vi "PW_LDA wrapper_PN.vi"(0 "PW_LDA control cluster":T2={"Block data directory"=path "C:/LDAPW data/x=140, y=0.79 10ms", "An samp. rate (Hz)"=5000.0, "PW sampling rate (Hz)"=10.0, "PW samples per block"=300, "High threshold (V)"=2.5, "An. data prefix"="Analogue_", "LDA data prefix"="LDA_", "PW data prefix"="PW_", "LDA arr. t. prefix"="LDA_arr_t_", "filename suffix"=".txt", "interp. method"=1, "PW hardware delay (s)"=0.00085, "PW timing TOF fraction (0..1)"=0.5, "- LDA V"=TRUE, "PW TOF prefix"="PW_TOF_", "- LDA U"=FALSE, "- PW"=FALSE, "format"="%.16f"} {"interp. method" items=["nearest", "linear", "spline", "cubic Hermite", "Lagrange"]}, 1 "Wrapper controls":T1={"N blocks"=20, "PW lag time start (s)"=0.0, "PW lag time finish (s)"=0.0, "PW lag time dt (s)"=0.002, "Desired lag time for stats (s)"=0.0, "stats order"=4, "PDF(T) or hist(F)"=TRUE, "Nbins U"=32, "Nbins V"=32, "Mean shift"=FALSE, "2nd comp."="v"}, 2 "Y pos":dbl) -> (13 "Y pos array":dbl[](array[numeric]), 14 "PW reverse flow factor":dbl=0.4096244131455399 format="%#_12g", 15 "All checksums okay":bool=TRUE, 16 "PW timeout fraction":dbl=0.012743125419181758, 17 "Rlag (m)":dbl[](array[numeric]), 18 "PW TOFmin cutoff fraction":dbl=0.001006036217303823, 19 "tlag (s)":dbl[](array[numeric]), 20 "Corr coeff. tau, U with PW lag time":dbl[](array[numeric])=[0.5572999061568849], 21 "Corr coeff. tau, V with PW lag time":dbl[](array[numeric])=[0.004298805974359152], 22 "Corr coeff. tau, UV with PW lag time":dbl[](array[numeric])=[-0.027234703441453165], 23 "Un-weighted stats":dbl[](array[numeric])=[0.43858590934936287, 0.0001041533801020402, 0.1463894386367247, -0.02457196354778752, 0.14225051082889828, -0.032883046319648, 0.02271213590005001, -0.030848260891795806, 0.020839430073599775, 1.6419504590373541, -0.017474933147796762, 0.26978335280499277, -0.029543622581726194, 0.2945426390265555, 0.03238576446532323, -0.16519945715490864, 0.09286281865203916, -0.1935441070795655, 0.050985700918232096, 6.779683511945926, -0.08550977449408034, 1.3778799507125228, -0.057532383884902095, 1.7073049444938453], 24 "Weighted stats":dbl[](array[numeric])=[0.29100923404306667, 0.003216404163501678, 0.14065168910394837, -0.0247339603407455, 0.13448157508469313, -0.024361823150874228, 0.02659079325503093, -0.029636337396151475, 0.03772631974230529, 1.334444078744411, -0.011181958349287136, 0.21516440173044252, -0.028718928576858992, 0.22755186986970175, 0.28082969747599357, -0.11371827995167888, 0.13120158382958494, -0.14829498580423525, 0.15080960131183163, 4.836358465323817, -0.08045155436100758, 0.9592749415988219, -0.10674333693310743, 1.117860734806738], 25 "Sync'd stats":dbl[](array[numeric])=[9.99808755719511, 0.30885001488943276, 0.007197594295384736, 0.0008830575291785714, 0.0942694270166445, -0.008369791241477553, 0.060882863617426265, -0.01639558282333675, 0.010021524505129425, -0.01919225938374916, -0.0007955532121171695, 1.081048634581646, -0.011113747117756345, 0.12842502593386193, 0.008713818152611364, 0.12343248218360064, 0.08560249872100657, -0.07896455364935291, 0.015579535060437296, -0.11211030347834718, -0.061338520775783154, 3.042693307359604, -0.042626691321700154, 0.4955635209260197, 0.12378215036474391, 0.6595145821544666, 4.519172989851708e-05, 5.91346531093378e-05, -0.00017430143164649768, -0.00021527961324126435, 0.019839799313372736, -0.000509583419996228, 0.002759758803593956, 0.0003530448602341623, 0.0027055215355820342, 0.0029382422465524904, -0.0014638561896802816, -0.00014761963473996917, -0.0025406145666271576, -0.0022637148963733722, 0.06455947587270858, -0.0015743835544541394, 0.012668430780602572, 0.004325247318679681, 0.016824152878582684, 0.025106752706962183, -0.015875686245146146, -0.006475981348485304, -0.02739532903645526, -0.026953861773836463, 0.0011723340448017852, -3.987256514453876e-05, 0.0001817240280323321, 3.3680352685292565e-06, 0.0001497262646277783, 0.0001415833115273109, -2.4675085527676877e-05, -1.8809858479403676e-05, -8.088971584500279e-05, -0.00010100909182132213, 0.002614922297046162, -9.514408147817417e-05, 0.000557542035268452, 0.00016469969685146263, 0.000676633068557077, 0.0008384732237052391, -0.0005110951840304789, -0.00037365314293173524, -0.0010324578366570894, -0.001198305036722039, 0.013265366110818869, 0.0002711809483820985, 0.0041643047012696185, 0.002418010535035754, 0.006215671063356672, 1.1217352583572477e-05, 6.344155160186447e-08, -7.664065504136946e-07, -2.129897917839301e-06, -5.306341303367024e-06, 0.0001195173198309039, -4.245802227303591e-06, 2.746649310552381e-05, 7.569471202211092e-06, 3.2191154509505075e-05, 1.0249380040762277e-05, -1.7041287981748652e-05, -2.1627786768005314e-05, -4.264139397480935e-05, -5.809335881508808e-05, 0.0005797512887398283, 3.959658308454404e-06, 0.00019648014213266728, 0.00010700455589582494, 0.00028675676203472286, 0.00018623104770989905, -0.0002861767092517544, -0.0002737802435507171, -0.0005887639922204611, -0.0007158972853763932, 1.6151006536221114e-05, -9.955295514799653e-07, 2.3778438821819195e-06, 3.3595543391506415e-07, 2.0535496541026416e-06, -5.444039236573482e-06, 3.5020997050138697e-07, -1.3997177108814566e-06, -1.6719714892314103e-06, -3.015766572187203e-06, 4.2187949113226374e-05, -1.9755684504406396e-06, 1.0753467015735944e-05, 4.47680139746371e-06, 1.4534458720814612e-05, -8.658088459848207e-06, -9.520921055642612e-06, -1.4596272866351805e-05, -2.6395769780853278e-05, -3.5099628626523324e-05, 0.0002370235802228167, 1.4637476763147469e-05, 0.00010148850801440133, 7.029378841714576e-05, 0.00016132576692576137], 26 "Total pre-sync LDA points":i32=44933, 27 "Total sync'd points":i32=5964)   [LabVIEW 2011]
uses:
  PW_LDA control cluster.ctl
  PW_LDA wrapper control cluster.ctl
  <vilib>/gmath/NI_Gmath.lvlib
  <vilib>/Analysis/NI_AALBase.lvlib
  <vilib>/Analysis/NI_AALPro.lvlib
panel:
  in  "Precision":i16=16
  out "PW lag time":dbl
  out "LDA V":dbl[](array[numeric])
  out "LDA U":dbl[](array[numeric])
  in  "Write lagged correls. file?":bool
  out "tlag(s) Rlag(m) tauU tauV tauUV":string="0.0000000000000000\t0.0000000000000000\t0.5572999061568848\t0.0042988059743592\t-0.0272347034414532\r\n"
  out "Lag time loop no.":i32=1
  out "Lag time loops to do":i32=1
  out "Block time pulse checksums":bool[](array[boolean])=[TRUE, TRUE, TRUE, TRUE, TRUE, TRUE, TRUE, TRUE, TRUE, TRUE, TRUE, TRUE, TRUE, TRUE, TRUE, TRUE, TRUE, TRUE, TRUE, TRUE]
  in  "Write raw numbers to file?":bool
  out "LDA orig. and sync'd U,V phase plot":cluster{"all rows":dbl[], "all rows":dbl[]}[](graph)
  out "PW, LDA_U, V, UV phase plot":cluster{"first row":dbl[], "yi":dbl[]}[](graph)
  out "Curr. block no.":i32=20
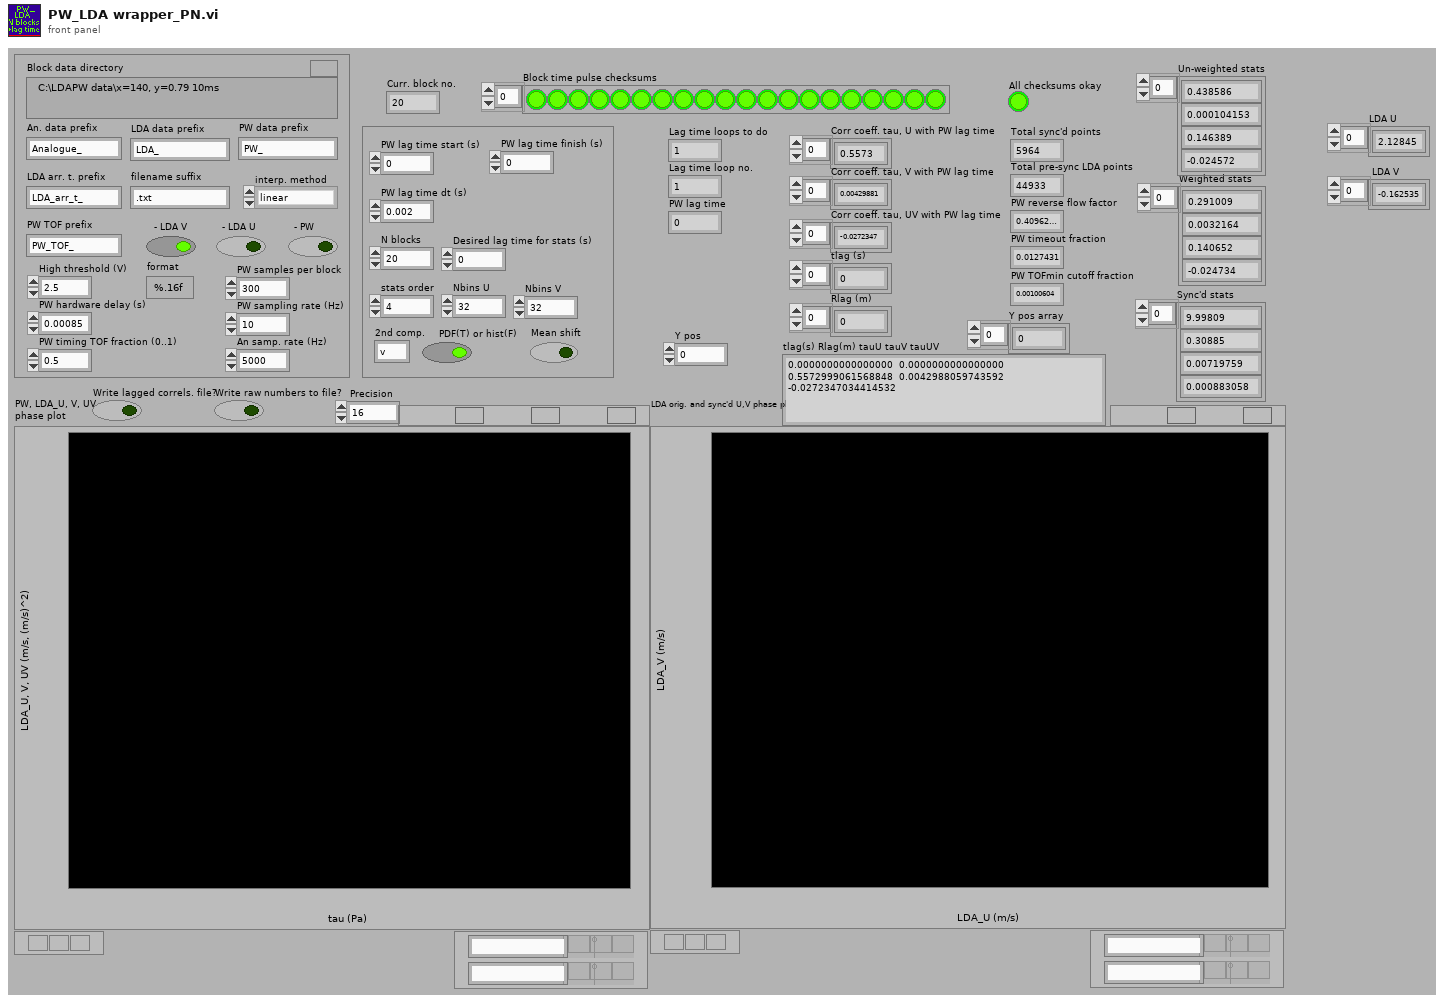
[diagram p1: front panel]
types:
  T1 = typedef "PW_LDA wrapper control cluster.ctl" = cluster{"N blocks":i32, "PW lag time start (s)":dbl, "PW lag time finish (s)":dbl, "PW lag time dt (s)":dbl, "Desired lag time for stats (s)":dbl, "stats order":i32, "PDF(T) or hist(F)":bool, "Nbins U":i32, "Nbins V":i32, "Mean shift":bool, "2nd comp.":string}
  T2 = typedef "PW_LDA control cluster.ctl" = cluster{"Block data directory":path, "An samp. rate (Hz)":dbl, "PW sampling rate (Hz)":dbl, "PW samples per block":i32, "High threshold (V)":dbl, "An. data prefix":string, "LDA data prefix":string, "PW data prefix":string, "LDA arr. t. prefix":string, "filename suffix":string, "interp. method":i32, "PW hardware delay (s)":dbl, "PW timing TOF fraction (0..1)":dbl, "- LDA V":bool, "PW TOF prefix":string, "- LDA U":bool, "- PW":bool, "format":string}
  T3 = enum16{"open", "replace", "create", "open or create", "replace or create", "replace or create with confirmation"}
  T4 = cluster{"sync'd LDA U":dbl[], "sync'd LDA U":dbl[]}
  T5 = cluster{"sync'd LDA U":dbl[], "sync'd LDA U":dbl[]}[]
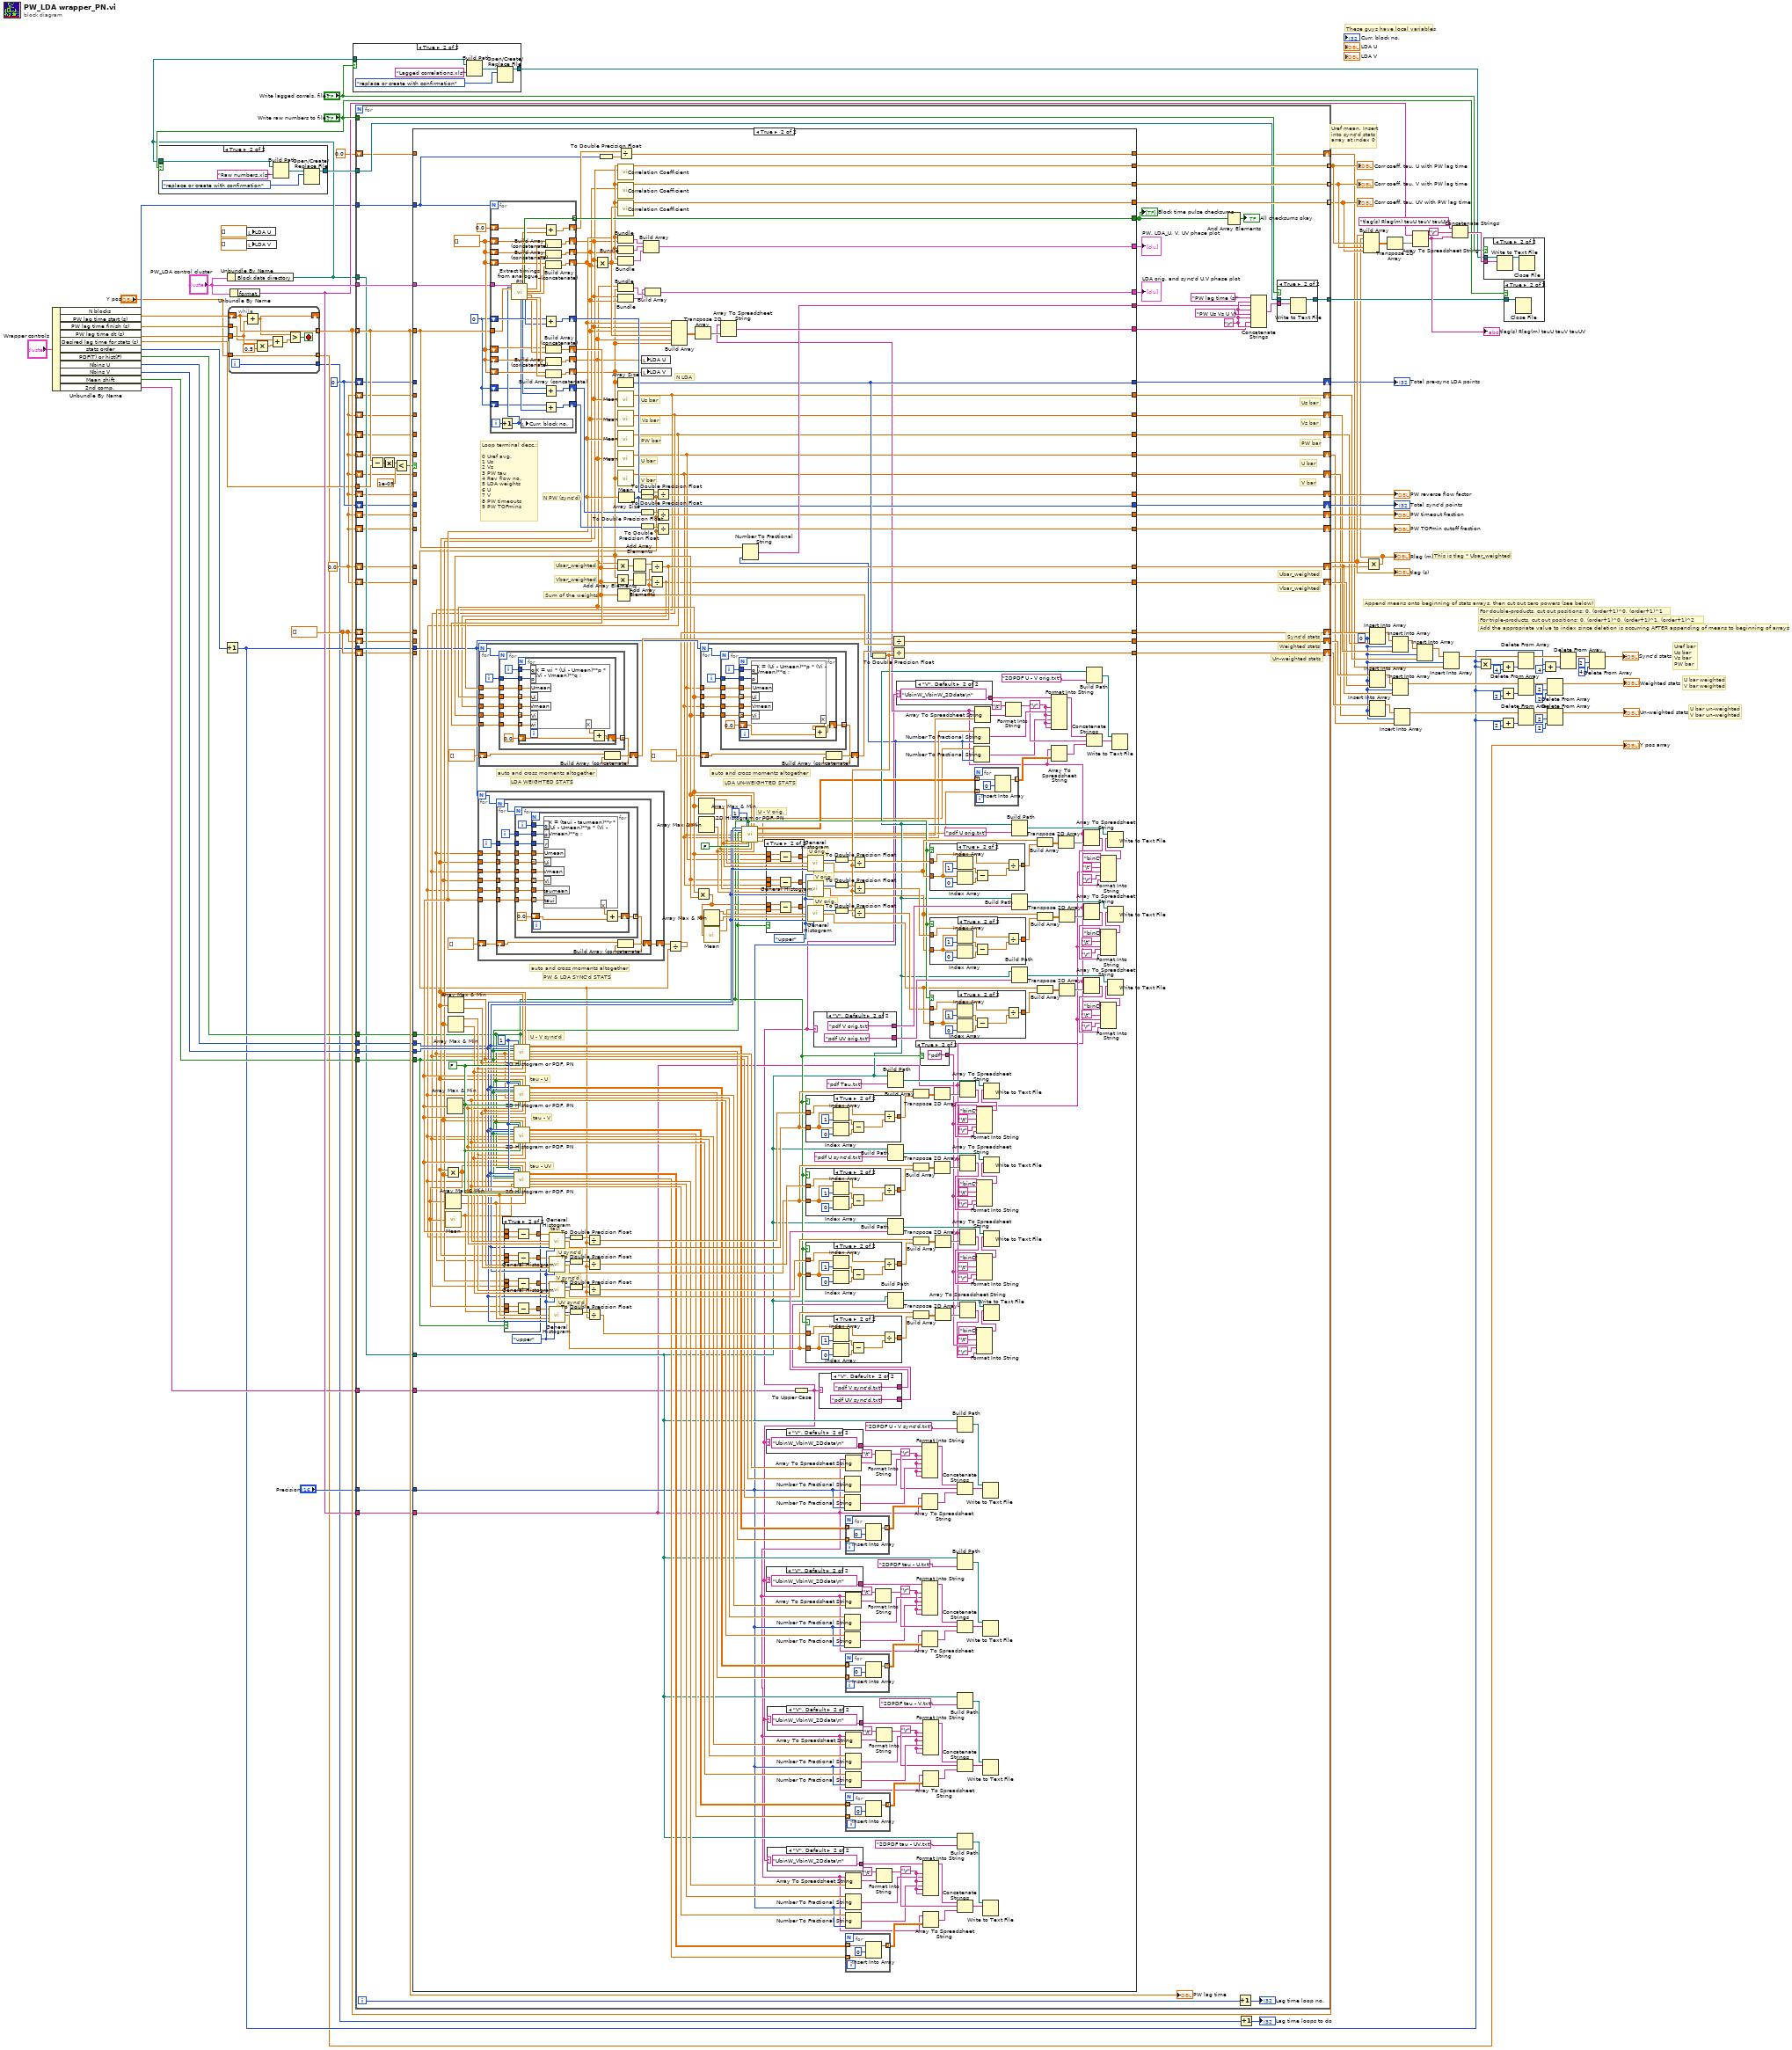
[diagram p0: block diagram]
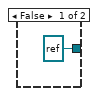
[diagram p3: hidden frame]
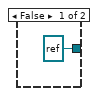
[diagram p4: hidden frame]
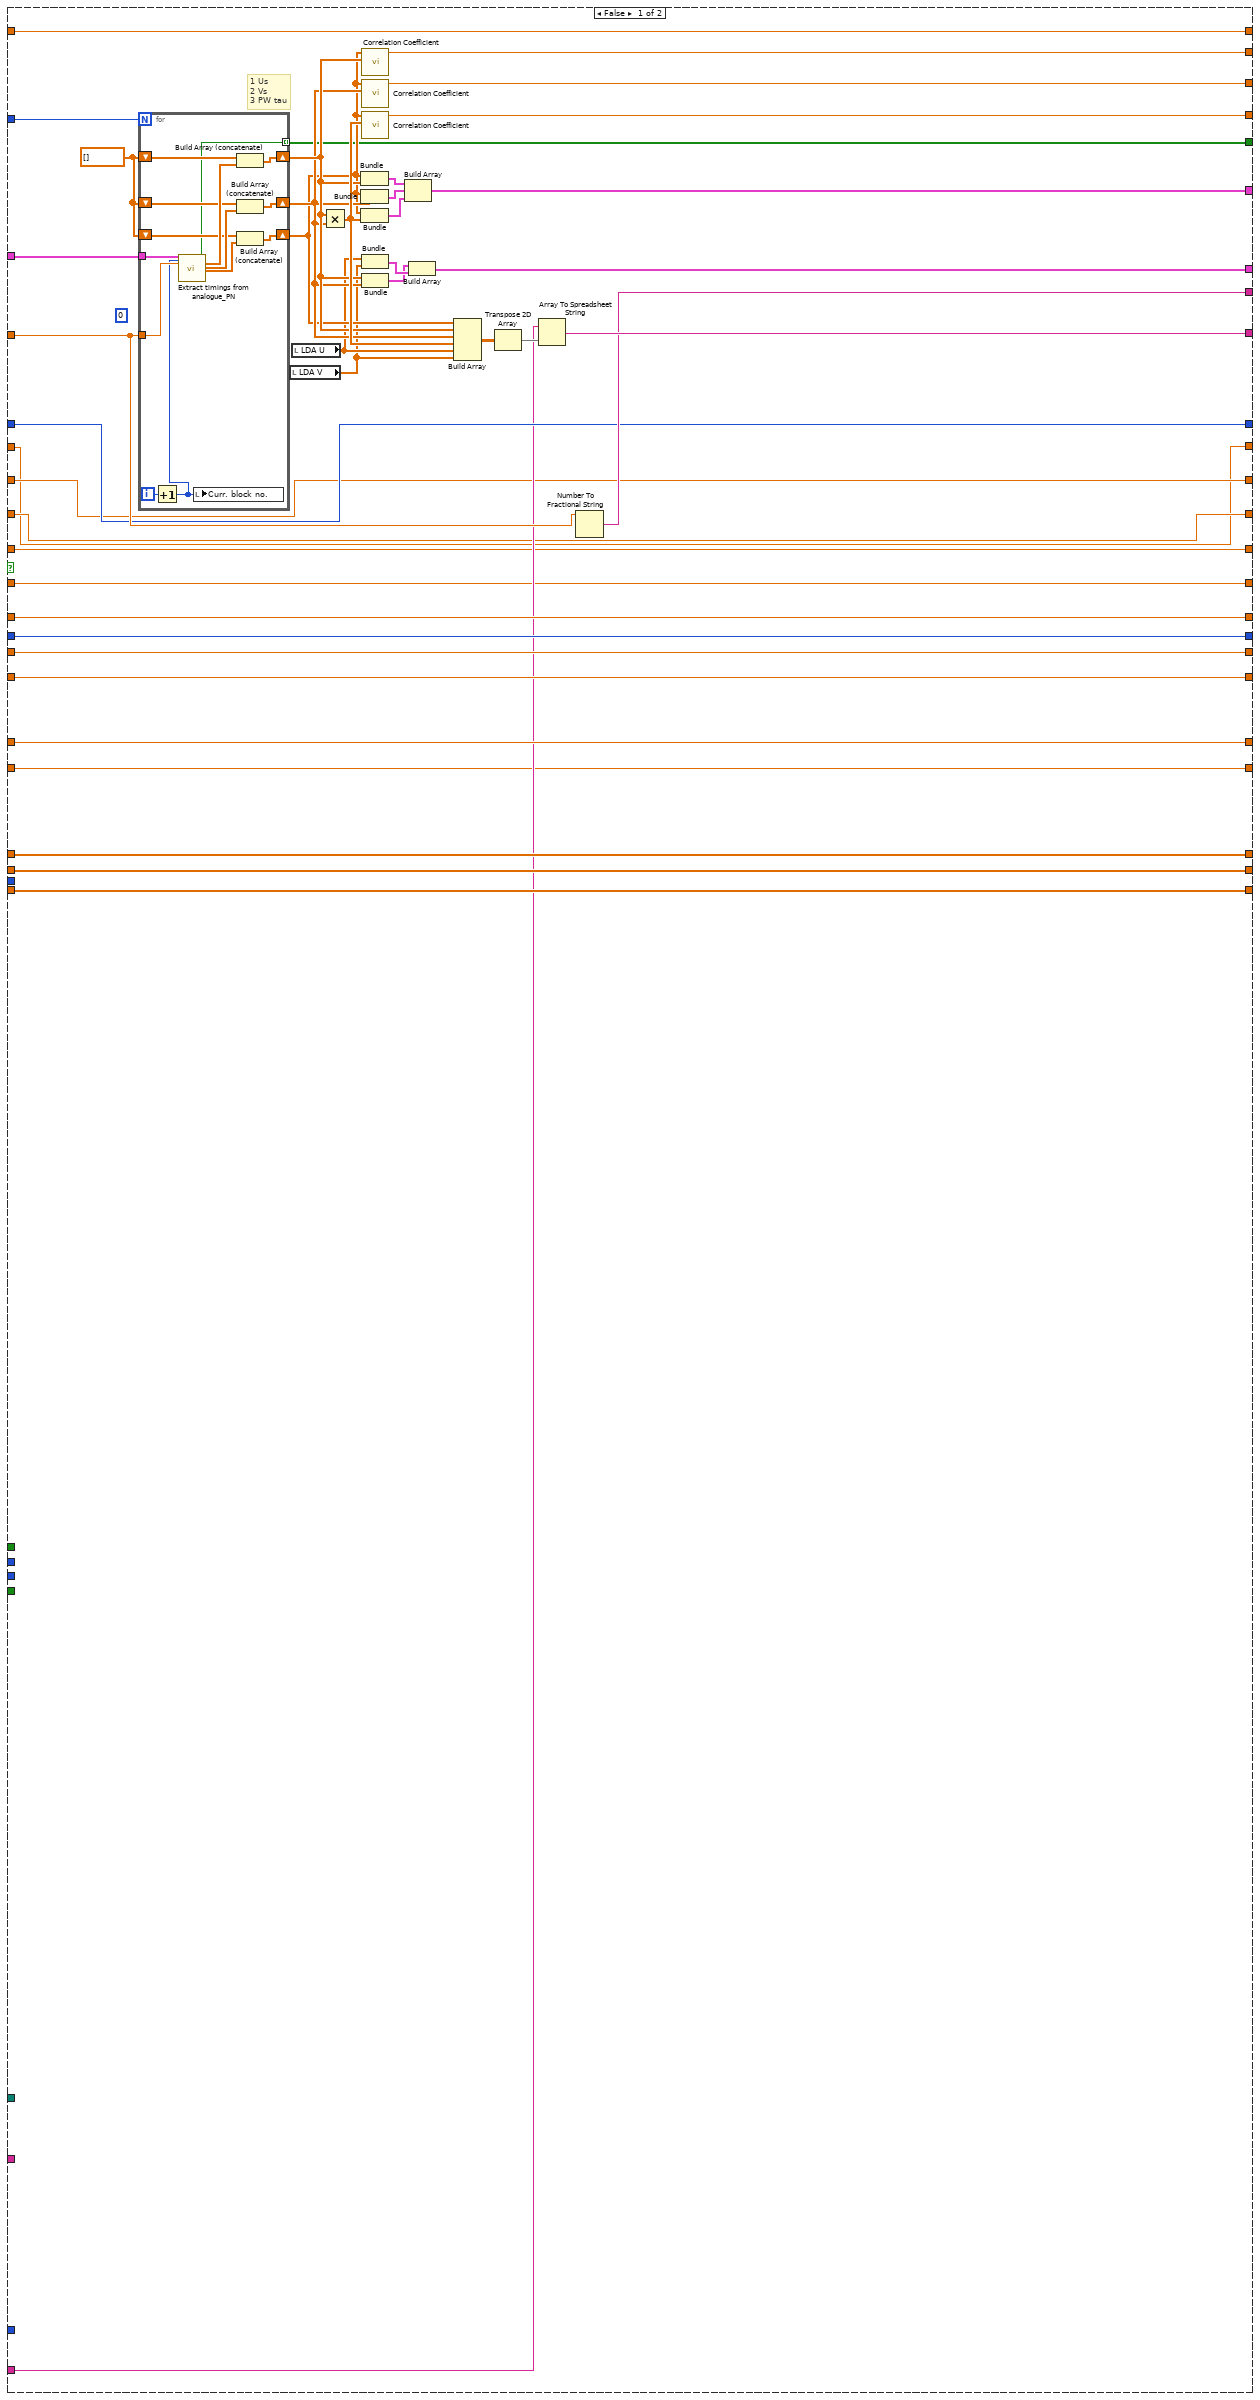
[diagram p7: hidden frame]
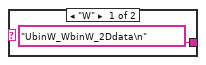
[diagram p8: hidden frame]
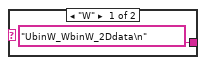
[diagram p9: hidden frame]
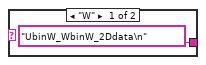
[diagram p10: hidden frame]
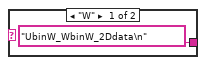
[diagram p11: hidden frame]
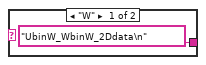
[diagram p12: hidden frame]
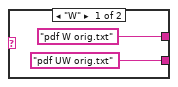
[diagram p13: hidden frame]
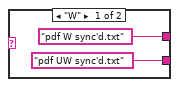
[diagram p18: hidden frame]
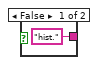
[diagram p19: hidden frame]
diagram:
  w5 = 0 ("index")
  w74 = dbl[] []
  w69 = 0
  w63 = 0.0
  # "Uref mean. Insert into sync'd stats array at index 0"
  # "Add the appropriate value to index since deletion is occurring AFTER appending of means to beginning of arrays"
  # "For triple-products, cut out positions: 0, (order+1)^0, (order+1)^1, (order+1)^2"
  # "For double-products, cut out positions: 0, (order+1)^0, (order+1)^1"
  # "U bar un-weighted\nV bar un-weighted"
  # "U bar weighted\nV bar weighted"
  # "Uref bar\nUs bar\nVs bar\nPW bar"
  # "Append means onto beginning of stats arrays, then cut out zero powers (see below)"
  # "This is tlag * Ubar_weighted"
  # "These guys have local variables"
  n1 = Unbundle By Name("Wrapper controls") -> ("N blocks"=w44:i32, "PW lag time start (s)"=w47:dbl, "PW lag time finish (s)"=w46:dbl, "PW lag time dt (s)"=w45:dbl, "Desired lag time for stats (s)"=w43:dbl, "stats order"=w37:i32, "PDF(T) or hist(F)"=w42:bool, "Nbins U"=w41:i32, "Nbins V"=w40:i32, "Mean shift"=w39:bool, "2nd comp."=w38:string)
  n2 = Increment(x=w37) -> (x+1=w12:i32)
  n3 = Unbundle By Name("PW_LDA control cluster") -> ("Block data directory"=w64:path)
  n4 = case shown="True" "Write raw numbers to file?" {
    tunnel: [refnum<file> refnum ("refnum out") w94] -> w82
    tunnel: w64 -> [_ w92]
    frame False {
    }
    frame True {
      n5 = Build Path(base path=w92, name or relative path="Raw numbers.xls") -> (appended path=w93:path)
      n6 = Open/Create/Replace File(file path (use dialog)=w93, operation (0:open)=T3."replace or create with confirmation") -> (refnum out=w94:refnum<file>)  [unwired: 1 in, 5 out]
    }
  }
  n7 = while {
    tunnel: w46 -> [w99]
    tunnel: w45 -> [w101]
    shift-right: [w103] -> _
    shift-left: w47 -> [w105]
    tunnel: [w105] -> w76 mode=indexing
    tunnel: [w104] -> w1
    tunnel: "Y pos" -> [w97]
    tunnel: [w97] -> w10 mode=indexing
    i -> [w104]
    stop <- w106 stop-if-true
    n8 = Add(x=w105, y=w101) -> (x+y=w103:dbl)
    n9 = Multiply(x=w101, y=0.5) -> (x*y=w100:dbl)
    n10 = Add(x=w99, y=w100) -> (x+y=w98:dbl)
    n11 = Greater?(x=w103, y=w98) -> (0:w106:bool)
  }
  "tlag (s)" <- w76
  "Y pos array" <- w10
  n12 = Unbundle By Name("PW_LDA control cluster") -> ("format"=w66:string)
  n13 = local write "LDA U"(dbl[] [] ("LDA U")) -> ()
  n14 = local write "LDA V"(dbl[] [] ("LDA V")) -> ()
  n15 = case shown="True" "Write lagged correls. file?" {
    tunnel: [refnum<file> refnum ("refnum out") w110] -> w80
    tunnel: w64 -> [_ w108]
    frame False {
    }
    frame True {
      n16 = Build Path(base path=w108, name or relative path="Lagged correlations.xls") -> (appended path=w109:path)
      n17 = Open/Create/Replace File(file path (use dialog)=w109, operation (0:open)=T3."replace or create with confirmation") -> (refnum out=w110:refnum<file>)  [unwired: 1 in, 5 out]
    }
  }
  n18 = for {
    tunnel: w44 -> [w179]
    tunnel: w76 -> [w164] mode=indexing
    tunnel: "Write raw numbers to file?" -> [w167]
    tunnel: [w178] -> w90 mode=indexing
    tunnel: [w177] -> w89 mode=indexing
    tunnel: [w176] -> w88 mode=indexing
    tunnel: w82 -> [w166]
    tunnel: [w168] -> w79
    tunnel: "PW_LDA control cluster" -> [w165]
    tunnel: w43 -> [w162]
    tunnel: w12 -> [w157]
    tunnel: w40 -> [w156]
    tunnel: w39 -> [w155]
    tunnel: w42 -> [w154]
    tunnel: w41 -> [w153]
    tunnel: w64 -> [w150]
    tunnel: "Precision" -> [w149]
    shift-right: [w158] -> w51
    shift-left: w63 -> [w143]
    shift-right: [w148] -> w61
    shift-left: w74 -> [w140]
    shift-right: [w147] -> w59
    shift-left: w74 -> [w139]
    shift-right: [w146] -> w56
    shift-left: w74 -> [w141]
    shift-right: [w152] -> w71
    shift-left: w63 -> [w135]
    shift-right: [w151] -> w70
    shift-left: w63 -> [w136]
    shift-right: [w142] -> w68
    shift-left: w69 -> [w132]
    shift-right: [w138] -> w73
    shift-left: w63 -> [w133]
    shift-right: [w137] -> w72
    shift-left: w69 -> [w134]
    tunnel: w66 -> [w131]
    shift-right: [w130] -> w54
    shift-left: w63 -> [w120]
    shift-right: [w129] -> w62
    shift-left: w63 -> [w121]
    shift-right: [w128] -> w53
    shift-left: w63 -> [w122]
    shift-right: [w127] -> w49
    shift-left: w63 -> [w123]
    shift-right: [w126] -> w50
    shift-left: w63 -> [w124]
    shift-right: [w125] -> w52
    shift-left: w63 -> [w118]
    tunnel: w38 -> [w119]
    shift-right: [w116] -> w4
    shift-left: 0.0 -> [w115]
    i -> [w114]
    w171 = "\r"
    # "Un-weighted stats"
    # "Weighted stats"
    # "Sync'd stats"
    # "Vbar_weighted"
    # "Ubar_weighted"
    # "V bar"
    # "U bar"
    # "PW bar"
    # "Vs bar"
    # "Us bar"
    n19 = Subtract(x=w164, y=w162) -> (x-y=w163:dbl)
    n20 = Absolute Value(x=w163) -> (abs(x)=w161:dbl)
    n21 = Less?(x=w161, y=1e-09) -> (x < y?=w159:bool)
    n22 = case shown="True" w159 {
      tunnel: w179 -> [w225 w241]
      tunnel: [w213 w526] -> w178
      tunnel: [w212 w525] -> w177
      tunnel: [w211 w524] -> w176
      tunnel: w164 -> [w204 w512]
      tunnel: [w209 w515] -> w117
      tunnel: [w192 w506] -> w142
      tunnel: [w193 w516] -> w138
      tunnel: [w194 w498] -> w137
      tunnel: [w197 w508] -> w147
      tunnel: [w208 w514] -> w170
      tunnel: [w207 w513] -> w169
      tunnel: w165 -> [w203 w511]
      tunnel: [w199 w507] -> w146
      tunnel: [w200 w505] -> w158
      tunnel: w157 -> [_ w497]
      tunnel: [w198 w396] -> w148
      tunnel: w156 -> [_ w472]
      tunnel: w155 -> [_ w458]
      tunnel: w154 -> [_ w335]
      tunnel: w153 -> [_ w473]
      tunnel: [w195 w489] -> w152
      tunnel: [w196 w488] -> w151
      tunnel: w150 -> [_ w265]
      tunnel: w149 -> [_ w259]
      tunnel: [w202 w258] -> w145
      tunnel: [w201 w257] -> w144
      tunnel: w143 -> [w200 _]
      tunnel: w141 -> [w199 _]
      tunnel: w140 -> [w198 _]
      tunnel: w139 -> [w197 _]
      tunnel: w136 -> [w196 _]
      tunnel: w135 -> [w195 _]
      tunnel: w134 -> [w194 _]
      tunnel: w133 -> [w193 _]
      tunnel: w132 -> [w192 _]
      tunnel: w131 -> [w191 w254]
      tunnel: [w185 w253] -> w130
      tunnel: [w186 w252] -> w129
      tunnel: [w187 w251] -> w128
      tunnel: [w188 w250] -> w127
      tunnel: [w189 w249] -> w126
      tunnel: [w190 w248] -> w125
      tunnel: w124 -> [w189 _]
      tunnel: w123 -> [w188 _]
      tunnel: w122 -> [w187 _]
      tunnel: w121 -> [w186 _]
      tunnel: w120 -> [w185 _]
      tunnel: w119 -> [_ w247]
      tunnel: w118 -> [w190 _]
      tunnel: [w184 w240] -> w116
      tunnel: w115 -> [w184 _]
      frame False {
        (unwired) 0 ("PW reverse flow samples")
        w210 = dbl[] [] ("sync'd LDA U")
        # "1 Us\n2 Vs\n3 PW tau"
        n23 = for {
          N: w225 -> [_]
          shift-right: [w236] -> w216
          shift-left: w210 -> [w238]
          shift-right: [w235] -> w215
          shift-left: w210 -> [w233]
          shift-right: [w232] -> w214
          shift-left: w210 -> [w230]
          tunnel: w204 -> [w227]
          tunnel: [w229] -> w209 mode=indexing
          tunnel: w203 -> [w228]
          i -> [w239]
          n24 = Increment(x=w239) -> (x+1=w226:i32)
          n25 = call "Extract timings from analogue_PN.vi"("PW_LDA control cluster"=w228, "Block no."=w226, "PW lag time (s)"=w227) -> ("valid bursts checksum status"=w229:bool, "sync'd LDA U"=w237:dbl[], "sync'd LDA V"=w234:dbl[], "PW tau"=w231:dbl[])  [unwired: 12 in, 9 out]
          n26 = local write "Curr. block no."(w226) -> ()
          n27 = Build Array (concatenate)(w238, w237) -> (w236:dbl[])
          n28 = Build Array (concatenate)(w233, w234) -> (w235:dbl[])
          n29 = Build Array (concatenate)(w230, w231) -> (w232:dbl[])
        }
        n30 = local read "LDA V"() -> (w205:dbl[])
        n31 = local read "LDA U"() -> (w206:dbl[])
        n32 = Multiply(x=w216, y=w215) -> (x*y=w217:dbl[])
        n33 = Bundle("sync'd LDA U"=w214, "sync'd LDA U"=w216) -> (w224:T4)  [unwired: 1 out]
        n34 = Bundle("sync'd LDA U"=w214, "sync'd LDA U"=w215) -> (w223:T4)  [unwired: 1 out]
        n35 = Bundle("sync'd LDA U"=w214, w217) -> (w222:cluster{"sync'd LDA U":dbl[], dbl[]})  [unwired: 1 out]
        n36 = call <vilib>:"Correlation Coefficient.vi"("Y"=w216, "X"=w214) -> ("correlation coefficient r"=w213:dbl)  [unwired: 9 out]
        n37 = call <vilib>:"Correlation Coefficient.vi"("Y"=w215, "X"=w214) -> ("correlation coefficient r"=w212:dbl)  [unwired: 9 out]
        n38 = call <vilib>:"Correlation Coefficient.vi"("Y"=w217, "X"=w214) -> ("correlation coefficient r"=w211:dbl)  [unwired: 9 out]
        n39 = Bundle("LDA U"=w206, "LDA V"=w205) -> (w221:cluster{"LDA U":dbl[], " LDA V":dbl[]})  [unwired: 1 out]
        n40 = Bundle("sync'd LDA U"=w216, "sync'd LDA U"=w215) -> (w220:T4)  [unwired: 1 out]
        n41 = Build Array(w224, w223, w222) -> (w202:T5)
        n42 = Build Array(w220, w221) -> (w201:cluster{"LDA U":dbl[], " LDA V":dbl[]}[])
        n43 = Build Array(w214, w216, w215, w217, w206, w205) -> (w219:dbl[][])
        n44 = Transpose 2D Array(2D array=w219) -> (transposed array=w218:dbl[][])
        n45 = Array To Spreadsheet String(array=w218, 3:w191) -> (spreadsheet string=w208:string)  [unwired: 1 out]
        n46 = Number To Fractional String(number=w204) -> (F-format string=w207:string)  [unwired: 3 out]
      }
      frame True {
        w476 = enum32{"lower", "upper"}."upper" ("inclusion")
        w479 = enum32{"lower", "upper"}."upper" ("inclusion")
        w276 = "\r"
        w296 = "\r"
        w306 = "\r"
        w332 = "\r"
        w343 = "\r"
        w495 = FALSE ("Interactive graph")
        w496 = 1 ("No. of blocks")
        w494 = 0 ("PW reverse flow samples")
        w523 = dbl[] [] ("sync'd LDA U")
        # "Sum of the weights"
        # "N PW (sync'd)"
        # "V bar"
        # "U bar"
        # "PW bar"
        # "Vs bar"
        # "Us bar"
        # "N LDA"
        # "UV orig."
        # "V orig."
        # "U orig."
        # "UV sync'd"
        # "V sync'd"
        # "U sync'd"
        # "tau"
        # "U - V orig."
        # "tau - UV"
        # "tau - V"
        # "tau - U"
        # "U - V sync'd"
        # "auto and cross moments altogether"
        # "auto and cross moments altogether"
        # "PW & LDA SYNC'd STATS"
        # "LDA UN-WEIGHTED STATS"
        # "LDA WEIGHTED STATS"
        # "Vbar_weighted"
        # "Ubar_weighted"
        # "auto and cross moments altogether"
        # "Loop terminal desc.:\n\n0 Uref avg.\n1 Us\n2 Vs\n3 PW tau\n4 Rev flow no.\n5 LDA weights\n6 U\n7 V\n8 PW timeouts\n9 PW TOFmins"
        n47 = for {
          N: w241 -> [_]
          shift-right: [w797] -> w465
          shift-left: w523 -> [w799]
          shift-right: [w796] -> w463
          shift-left: w523 -> [w794]
          shift-right: [w793] -> w467
          shift-left: w523 -> [w791]
          shift-right: [w790] -> w256
          shift-left: w523 -> [w789]
          shift-right: [w787] -> w255
          shift-left: w523 -> [w785]
          tunnel: w512 -> [w776]
          tunnel: [w784] -> w515 mode=indexing
          shift-right: [w782] -> w510
          shift-left: w523 -> [w781]
          shift-right: [w780] -> w518
          shift-left: w494 -> [w778]
          tunnel: w511 -> [w777]
          shift-right: [w772] -> w490
          shift-left: w494 -> [w770]
          shift-right: [w771] -> w491
          shift-left: w494 -> [w769]
          shift-right: [w767] -> w242
          shift-left: 0.0 -> [w766]
          i -> [w800]
          n48 = Increment(x=w800) -> (x+1=w774:i32)
          n49 = call "Extract timings from analogue_PN.vi"("PW_LDA control cluster"=w777, "Block no."=w774, "PW lag time (s)"=w776) -> ("No. of PW <TOFmin"=w773:i32, "Uref block avg."=w768:dbl, "No. of PW timeouts"=w775:i32, "valid bursts checksum status"=w784:bool, "PW reverse flow samples"=w779:i32, "sync'd LDA U"=w798:dbl[], "sync'd LDA V"=w795:dbl[], "PW tau"=w792:dbl[], "LDA weights"=w783:dbl[], "LDA U"=w788:dbl[], "LDA V"=w786:dbl[])  [unwired: 12 in, 2 out]
          n50 = local write "Curr. block no."(w774) -> ()
          n51 = Add(x=w766, y=w768) -> (x+y=w767:dbl)
          n52 = Add(x=w778, y=w779) -> (x+y=w780:i32)
          n53 = Add(x=w770, y=w775) -> (x+y=w772:i32)
          n54 = Add(x=w769, y=w773) -> (x+y=w771:i32)
          n55 = Build Array (concatenate)(w799, w798) -> (w797:dbl[])
          n56 = Build Array (concatenate)(w794, w795) -> (w796:dbl[])
          n57 = Build Array (concatenate)(w791, w792) -> (w793:dbl[])
          n58 = Build Array (concatenate)(w781, w783) -> (w782:dbl[])
          n59 = Build Array (concatenate)(w789, w788) -> (w790:dbl[])
          n60 = Build Array (concatenate)(w785, w786) -> (w787:dbl[])
        }
        n61 = Multiply(x=w465, y=w463) -> (x*y=w461:dbl[])
        n62 = Array Max & Min(array=w461) -> (max value=w477:dbl, min value=w478:dbl)  [unwired: 2 out]
        n63 = call <vilib>:"Mean.vi"("X"=w461) -> ("mean"=w459:dbl)  [unwired: 1 out]
        n64 = Array Max & Min(array=w467) -> (max value=w485:dbl, min value=w484:dbl)  [unwired: 2 out]
        n65 = Array Max & Min(array=w465) -> (max value=w482:dbl, min value=w483:dbl)  [unwired: 2 out]
        n66 = Array Max & Min(array=w463) -> (max value=w480:dbl, min value=w481:dbl)  [unwired: 2 out]
        n67 = Multiply(x=w465, y=w463) -> (x*y=w527:dbl[])
        n68 = To Double Precision Float(number=w241) -> (double precision float=w243:dbl)
        n69 = Multiply(x=w256, y=w510) -> (x*y=w522:dbl[])
        n70 = Multiply(x=w255, y=w510) -> (x*y=w519:dbl[])
        n71 = Add Array Elements(numeric array=w510) -> (sum=w509:dbl)
        n72 = Bundle("sync'd LDA U"=w467, "sync'd LDA U"=w465) -> (w534:T4)  [unwired: 1 out]
        n73 = Bundle("sync'd LDA U"=w467, "sync'd LDA U"=w463) -> (w533:T4)  [unwired: 1 out]
        n74 = Bundle("sync'd LDA U"=w467, w527) -> (w532:cluster{"sync'd LDA U":dbl[], dbl[]})  [unwired: 1 out]
        n75 = Divide(x=w242, y=w243) -> (x/y=w240:dbl)
        n76 = call <vilib>:"Correlation Coefficient.vi"("Y"=w465, "X"=w467) -> ("correlation coefficient r"=w526:dbl)  [unwired: 9 out]
        n77 = call <vilib>:"Correlation Coefficient.vi"("Y"=w463, "X"=w467) -> ("correlation coefficient r"=w525:dbl)  [unwired: 9 out]
        n78 = call <vilib>:"Correlation Coefficient.vi"("Y"=w527, "X"=w467) -> ("correlation coefficient r"=w524:dbl)  [unwired: 9 out]
        n79 = Bundle("sync'd LDA U"=w256, "sync'd LDA U"=w255) -> (w531:T4)  [unwired: 1 out]
        n80 = Bundle("sync'd LDA U"=w465, "sync'd LDA U"=w463) -> (w530:T4)  [unwired: 1 out]
        n81 = Array Size(array=w255) -> (size(s)=w506:i32)
        n82 = call <vilib>:"Mean.vi"("X"=w465) -> ("mean"=w253:dbl)  [unwired: 1 out]
        n83 = call <vilib>:"Mean.vi"("X"=w463) -> ("mean"=w252:dbl)  [unwired: 1 out]
        n84 = call "2D Histogram or PDF, PN.vi"("Nbins U"=w473, "Nbins V"=w472, "Mean shift"=w458, "Umean"=w253, "Vmean"=w252, "Umax"=w482, "No. of blocks"=w496, "Umin"=w483, "PDF"=w335, "Interactive graph"=w495, "V"=w463, "Vmax"=w480, "U"=w465, "Vmin"=w481) -> ("2D histogram or PDF"=w338:dbl[][], "U bin centre vals."=w339:dbl[], "V bin centre vals."=w340:dbl[], "UbinWidth"=w337:dbl, "VbinWidth"=w336:dbl)  [unwired: 1 out]
        n85 = call <vilib>:"Mean.vi"("X"=w467) -> ("mean"=w251:dbl)  [unwired: 1 out]
        n86 = for {
          N: w497 -> [w675]
          shift-right: [w673] -> w499
          shift-left: dbl[] [] -> [w674]
          tunnel: w467 -> [w672]
          tunnel: w251 -> [w671]
          tunnel: w465 -> [w670]
          tunnel: w463 -> [w669]
          tunnel: w253 -> [w668]
          tunnel: w252 -> [w667]
          i -> [w666]
          n87 = for {
            N: w675 -> [w680]
            tunnel: w670 -> [w687]
            tunnel: w669 -> [w686]
            tunnel: w667 -> [w685]
            tunnel: w668 -> [w684]
            shift-right: [w682] -> w673
            shift-left: w674 -> [w683]
            tunnel: w666 -> [w679]
            tunnel: w672 -> [w677]
            tunnel: w671 -> [w676]
            i -> [w678]
            n88 = for {
              N: w680 -> [_]
              tunnel: w684 -> [w698]
              tunnel: w687 -> [w697]
              tunnel: [w692] -> w681 mode=indexing
              tunnel: w685 -> [w695]
              tunnel: w686 -> [w694]
              tunnel: w678 -> [w693]
              tunnel: w679 -> [w691]
              tunnel: w677 -> [w690]
              tunnel: w676 -> [w689]
              i -> [w688]
              n89 = for {
                tunnel: w698 -> [w710]
                tunnel: w697 -> [w709] mode=indexing
                shift-right: [w707] -> w692
                shift-left: 0.0 -> [w706]
                tunnel: w688 -> [w703]
                tunnel: w695 -> [w705]
                tunnel: w694 -> [w704] mode=indexing
                tunnel: w693 -> [w702]
                tunnel: w691 -> [w701]
                tunnel: w690 -> [w700] mode=indexing
                tunnel: w689 -> [w699]
                n90 = formula code="X = (taui - taumean)**r * (Ui - Umean)**p * (Vi - Vmean)**q ;"("Umean"=w710, "Ui"=w709, "p"=w702, "Vi"=w704, "Vmean"=w705, "q"=w703, "r"=w701, "taumean"=w699, "taui"=w700) -> ("X"=w708:dbl)
                n91 = Add(x=w708, y=w706) -> (x+y=w707:dbl)
              }
            }
            n92 = Build Array (concatenate)(w683, w681) -> (w682:dbl[])
          }
        }
        n93 = case shown="True" w458 {
          tunnel: w467 -> [w653 w665]
          tunnel: [w653 w664] -> w466
          tunnel: w251 -> [_ w663]
          tunnel: w465 -> [w652 w662]
          tunnel: [w652 w661] -> w464
          tunnel: w253 -> [_ w660]
          tunnel: w463 -> [w651 w659]
          tunnel: [w651 w658] -> w462
          tunnel: w252 -> [_ w657]
          tunnel: w461 -> [w650 w656]
          tunnel: [w650 w655] -> w460
          tunnel: w459 -> [_ w654]
          frame False {
          }
          frame True {
            n94 = Subtract(x=w665, y=w663) -> (x-y=w664:dbl[])
            n95 = Subtract(x=w662, y=w660) -> (x-y=w661:dbl[])
            n96 = Subtract(x=w659, y=w657) -> (x-y=w658:dbl[])
            n97 = Subtract(x=w656, y=w654) -> (x-y=w655:dbl[])
          }
        }
        n98 = call "2D Histogram or PDF, PN.vi"("Nbins U"=w473, "Nbins V"=w472, "Mean shift"=w458, "Umean"=w251, "Vmean"=w253, "Umax"=w485, "No. of blocks"=w496, "Umin"=w484, "PDF"=w335, "Interactive graph"=w495, "V"=w465, "Vmax"=w482, "U"=w467, "Vmin"=w483) -> ("2D histogram or PDF"=w318:dbl[][], "U bin centre vals."=w317:dbl[], "V bin centre vals."=w321:dbl[], "UbinWidth"=w320:dbl, "VbinWidth"=w319:dbl)  [unwired: 1 out]
        n99 = call "2D Histogram or PDF, PN.vi"("Nbins U"=w473, "Nbins V"=w472, "Mean shift"=w458, "Umean"=w251, "Vmean"=w252, "Umax"=w485, "No. of blocks"=w496, "Umin"=w484, "PDF"=w335, "Interactive graph"=w495, "V"=w463, "Vmax"=w480, "U"=w467, "Vmin"=w481) -> ("2D histogram or PDF"=w300:dbl[][], "U bin centre vals."=w299:dbl[], "V bin centre vals."=w303:dbl[], "UbinWidth"=w302:dbl, "VbinWidth"=w301:dbl)  [unwired: 1 out]
        n100 = call "2D Histogram or PDF, PN.vi"("Nbins U"=w473, "Nbins V"=w472, "Mean shift"=w458, "Umean"=w251, "Vmean"=w459, "Umax"=w485, "No. of blocks"=w496, "Umin"=w484, "PDF"=w335, "Interactive graph"=w495, "V"=w461, "Vmax"=w477, "U"=w467, "Vmin"=w478) -> ("2D histogram or PDF"=w282:dbl[][], "U bin centre vals."=w281:dbl[], "V bin centre vals."=w285:dbl[], "UbinWidth"=w284:dbl, "VbinWidth"=w283:dbl)  [unwired: 1 out]
        n101 = call <vilib>:"General Histogram.vi"("X"=w466, "max"=w485, "min"=w484, "# bins"=w473, "inclusion"=w479) -> ("Histogram"=w424:i32[], "Axis"=w402:dbl[])  [unwired: 1 in, 8 out]
        n102 = call <vilib>:"General Histogram.vi"("X"=w464, "max"=w482, "min"=w483, "# bins"=w473, "inclusion"=w479) -> ("Histogram"=w418:i32[], "Axis"=w413:dbl[])  [unwired: 1 in, 8 out]
        n103 = call <vilib>:"General Histogram.vi"("X"=w462, "max"=w480, "min"=w481, "# bins"=w472, "inclusion"=w479) -> ("Histogram"=w419:i32[], "Axis"=w397:dbl[])  [unwired: 1 in, 8 out]
        n104 = call <vilib>:"General Histogram.vi"("X"=w460, "max"=w477, "min"=w478, "# bins"=w472, "inclusion"=w479) -> ("Histogram"=w420:i32[], "Axis"=w416:dbl[])  [unwired: 1 in, 8 out]
        n105 = To Double Precision Float(number=w424) -> (double precision float=w425:dbl[])
        n106 = To Double Precision Float(number=w418) -> (double precision float=w423:dbl[])
        n107 = To Double Precision Float(number=w419) -> (double precision float=w422:dbl[])
        n108 = To Double Precision Float(number=w420) -> (double precision float=w421:dbl[])
        n109 = call <vilib>:"Mean.vi"("X"=w256) -> ("mean"=w250:dbl)  [unwired: 1 out]
        n110 = call <vilib>:"Mean.vi"("X"=w255) -> ("mean"=w249:dbl)  [unwired: 1 out]
        n111 = Array Size(array=w467) -> (size(s)=w498:i32)
        n112 = Add Array Elements(numeric array=w522) -> (sum=w520:dbl)
        n113 = Add Array Elements(numeric array=w519) -> (sum=w521:dbl)
        n114 = To Double Precision Float(number=w518) -> (double precision float=w517:dbl)
        n115 = To Double Precision Float(number=w498) -> (double precision float=w245:dbl)
        n116 = Divide(x=w425, y=w245) -> (x/y=w403:dbl[])
        n117 = Divide(x=w423, y=w245) -> (x/y=w414:dbl[])
        n118 = Divide(x=w422, y=w245) -> (x/y=w415:dbl[])
        n119 = Divide(x=w421, y=w245) -> (x/y=w417:dbl[])
        n120 = To Double Precision Float(number=w490) -> (double precision float=w492:dbl)
        n121 = To Double Precision Float(number=w491) -> (double precision float=w493:dbl)
        n122 = local write "LDA U"(w256) -> ()
        n123 = local write "LDA V"(w255) -> ()
        n124 = Build Array(w534, w533, w532) -> (w258:T5)
        n125 = Build Array(w530, w531) -> (w257:T5)
        n126 = Divide(x=w520, y=w509) -> (x/y=w505:dbl)
        n127 = Divide(x=w521, y=w509) -> (x/y=w248:dbl)
        n128 = for {
          N: w497 -> [w739]
          tunnel: w256 -> [w746]
          tunnel: w255 -> [w745]
          tunnel: w248 -> [w744]
          tunnel: w505 -> [w743]
          shift-right: [w741] -> w501
          shift-left: dbl[] [] -> [w742]
          tunnel: w510 -> [w738]
          i -> [w737]
          n129 = for {
            N: w739 -> [_]
            tunnel: w743 -> [w755]
            tunnel: w746 -> [w754]
            tunnel: [w749] -> w740 mode=indexing
            tunnel: w744 -> [w752]
            tunnel: w745 -> [w751]
            tunnel: w737 -> [w750]
            tunnel: w738 -> [w748]
            i -> [w747]
            n130 = for {
              tunnel: w755 -> [w765]
              tunnel: w754 -> [w764] mode=indexing
              shift-right: [w762] -> w749
              shift-left: 0.0 -> [w761]
              tunnel: w747 -> [w758]
              tunnel: w752 -> [w760]
              tunnel: w751 -> [w759] mode=indexing
              tunnel: w750 -> [w757]
              tunnel: w748 -> [w756] mode=indexing
              n131 = formula code="X = wi * (Ui - Umean)**p * (Vi - Vmean)**q ;"("Umean"=w765, "Ui"=w764, "p"=w757, "Vi"=w759, "Vmean"=w760, "q"=w758, "wi"=w756) -> ("X"=w763:dbl)
              n132 = Add(x=w763, y=w761) -> (x+y=w762:dbl)
            }
          }
          n133 = Build Array (concatenate)(w742, w740) -> (w741:dbl[])
        }
        n134 = Divide(x=w517, y=w245) -> (x/y=w516:dbl)
        n135 = Divide(x=w492, y=w245) -> (x/y=w489:dbl)
        n136 = Divide(x=w493, y=w245) -> (x/y=w488:dbl)
        n137 = Divide(x=w499, y=w245) -> (x/y=w396:dbl[])
        n138 = Build Array(w467, w465, w463, w527, w256, w255) -> (w529:dbl[][])
        n139 = Transpose 2D Array(2D array=w529) -> (transposed array=w528:dbl[][])
        n140 = Multiply(x=w256, y=w255) -> (x*y=w454:dbl[])
        n141 = Array Max & Min(array=w256) -> (max value=w474:dbl, min value=w475:dbl)  [unwired: 2 out]
        n142 = Array Max & Min(array=w255) -> (max value=w470:dbl, min value=w471:dbl)  [unwired: 2 out]
        n143 = for {
          N: w497 -> [w712]
          tunnel: w256 -> [w719]
          tunnel: w255 -> [w718]
          tunnel: w249 -> [w717]
          tunnel: w250 -> [w716]
          shift-right: [w714] -> w500
          shift-left: dbl[] [] -> [w715]
          i -> [w711]
          n144 = for {
            N: w712 -> [_]
            tunnel: w716 -> [w727]
            tunnel: w719 -> [w726]
            tunnel: [w721] -> w713 mode=indexing
            tunnel: w717 -> [w724]
            tunnel: w718 -> [w723]
            tunnel: w711 -> [w722]
            i -> [w720]
            n145 = for {
              tunnel: w727 -> [w736]
              tunnel: w726 -> [w735] mode=indexing
              shift-right: [w733] -> w721
              shift-left: 0.0 -> [w732]
              tunnel: w720 -> [w729]
              tunnel: w724 -> [w731]
              tunnel: w723 -> [w730] mode=indexing
              tunnel: w722 -> [w728]
              n146 = formula code="X = (Ui - Umean)**p * (Vi - Vmean)**q ;"("Umean"=w736, "Ui"=w735, "p"=w728, "Vi"=w730, "Vmean"=w731, "q"=w729) -> ("X"=w734:dbl)
              n147 = Add(x=w734, y=w732) -> (x+y=w733:dbl)
            }
          }
          n148 = Build Array (concatenate)(w715, w713) -> (w714:dbl[])
        }
        n149 = Array Max & Min(array=w454) -> (max value=w469:dbl, min value=w468:dbl)  [unwired: 2 out]
        n150 = call <vilib>:"Mean.vi"("X"=w454) -> ("mean"=w453:dbl)  [unwired: 1 out]
        n151 = Array To Spreadsheet String(array=w528, 3:w254) -> (spreadsheet string=w514:string)  [unwired: 1 out]
        n152 = call "2D Histogram or PDF, PN.vi"("Nbins U"=w473, "Nbins V"=w472, "Mean shift"=w458, "Umean"=w250, "Vmean"=w249, "Umax"=w474, "No. of blocks"=1, "Umin"=w475, "PDF"=w335, "Interactive graph"=FALSE, "V"=w255, "Vmax"=w470, "U"=w256, "Vmin"=w471) -> ("2D histogram or PDF"=w263:dbl[][], "U bin centre vals."=w262:dbl[], "V bin centre vals."=w264:dbl[], "UbinWidth"=w261:dbl, "VbinWidth"=w260:dbl)  [unwired: 1 out]
        n153 = Number To Fractional String(number=w512, precision (6)=w259) -> (F-format string=w513:string)  [unwired: 2 out]
        n154 = case shown="True" w458 {
          tunnel: w256 -> [w640 w649]
          tunnel: [w640 w648] -> w457
          tunnel: w250 -> [_ w647]
          tunnel: w255 -> [w639 w646]
          tunnel: [w639 w645] -> w456
          tunnel: w249 -> [_ w644]
          tunnel: w454 -> [w638 w643]
          tunnel: [w638 w642] -> w455
          tunnel: w453 -> [_ w641]
          frame False {
          }
          frame True {
            n155 = Subtract(x=w649, y=w647) -> (x-y=w648:dbl[])
            n156 = Subtract(x=w646, y=w644) -> (x-y=w645:dbl[])
            n157 = Subtract(x=w643, y=w641) -> (x-y=w642:dbl[])
          }
        }
        n158 = To Upper Case(1:w247) -> (0:w246:string)
        n159 = case shown="\"V\", Default" w246 {
          tunnel: ["UbinW_WbinW_2Ddata\n" ("initial string") "UbinW_VbinW_2Ddata\n" ("initial string")] -> w342
          frame "W" {
          }
          frame "V", Default {
          }
        }
        n160 = case shown="\"V\", Default" w246 {
          tunnel: ["UbinW_WbinW_2Ddata\n" ("initial string") "UbinW_VbinW_2Ddata\n" ("initial string")] -> w333
          frame "W" {
          }
          frame "V", Default {
          }
        }
        n161 = case shown="\"V\", Default" w246 {
          tunnel: ["UbinW_WbinW_2Ddata\n" ("initial string") "UbinW_VbinW_2Ddata\n" ("initial string")] -> w305
          frame "W" {
          }
          frame "V", Default {
          }
        }
        n162 = case shown="\"V\", Default" w246 {
          tunnel: ["UbinW_WbinW_2Ddata\n" ("initial string") "UbinW_VbinW_2Ddata\n" ("initial string")] -> w297
          frame "W" {
          }
          frame "V", Default {
          }
        }
        n163 = case shown="True" w335 {
          tunnel: [w596 w598] -> w407
          tunnel: w403 -> [w596 w599]
          tunnel: w402 -> [_ w603]
          frame False {
          }
          frame True {
            n164 = Index Array(array=w603, index=1) -> (element=w601:dbl)
            n165 = Index Array(array=w603, index=0) -> (element=w600:dbl)
            n166 = Subtract(x=w601, y=w600) -> (x-y=w597:dbl)
            n167 = Divide(x=w599, y=w597) -> (x/y=w598:dbl[])
          }
        }
        n168 = case shown="True" w335 {
          tunnel: [w629 w631] -> w449
          tunnel: w414 -> [w629 w632]
          tunnel: w413 -> [_ w636]
          frame False {
          }
          frame True {
            n169 = Index Array(array=w636, index=1) -> (element=w634:dbl)
            n170 = Index Array(array=w636, index=0) -> (element=w633:dbl)
            n171 = Subtract(x=w634, y=w633) -> (x-y=w630:dbl)
            n172 = Divide(x=w632, y=w630) -> (x/y=w631:dbl[])
          }
        }
        n173 = case shown="True" w335 {
          tunnel: [w620 w623] -> w448
          tunnel: w415 -> [w620 w624]
          tunnel: w397 -> [_ w621]
          frame False {
          }
          frame True {
            n174 = Index Array(array=w621, index=1) -> (element=w626:dbl)
            n175 = Index Array(array=w621, index=0) -> (element=w625:dbl)
            n176 = Subtract(x=w626, y=w625) -> (x-y=w622:dbl)
            n177 = Divide(x=w624, y=w622) -> (x/y=w623:dbl[])
          }
        }
        n178 = case shown="True" w335 {
          tunnel: [w611 w613] -> w442
          tunnel: w417 -> [w611 w614]
          tunnel: w416 -> [_ w618]
          frame False {
          }
          frame True {
            n179 = Index Array(array=w618, index=1) -> (element=w616:dbl)
            n180 = Index Array(array=w618, index=0) -> (element=w615:dbl)
            n181 = Subtract(x=w616, y=w615) -> (x-y=w612:dbl)
            n182 = Divide(x=w614, y=w612) -> (x/y=w613:dbl[])
          }
        }
        n183 = call <vilib>:"General Histogram.vi"("X"=w457, "max"=w474, "min"=w475, "# bins"=w473, "inclusion"=w476) -> ("Histogram"=w363:i32[], "Axis"=w354:dbl[])  [unwired: 1 in, 8 out]
        n184 = call <vilib>:"General Histogram.vi"("X"=w456, "max"=w470, "min"=w471, "# bins"=w472, "inclusion"=w476) -> ("Histogram"=w361:i32[], "Axis"=w280:dbl[])  [unwired: 1 in, 8 out]
        n185 = call <vilib>:"General Histogram.vi"("X"=w455, "max"=w469, "min"=w468, "# bins"=w472, "inclusion"=w476) -> ("Histogram"=w362:i32[], "Axis"=w279:dbl[])  [unwired: 1 in, 8 out]
        n186 = case shown="\"V\", Default" w246 {
          tunnel: ["pdf W orig.txt" ("string") "pdf V orig.txt" ("string")] -> w393
          tunnel: ["pdf UW orig.txt" ("string") "pdf UV orig.txt" ("string")] -> w394
          frame "W" {
          }
          frame "V", Default {
          }
        }
        n187 = case shown="\"V\", Default" w246 {
          tunnel: ["pdf W sync'd.txt" ("string") "pdf V sync'd.txt" ("string")] -> w401
          tunnel: ["pdf UW sync'd.txt" ("string") "pdf UV sync'd.txt" ("string")] -> w400
          frame "W" {
          }
          frame "V", Default {
          }
        }
        n188 = To Double Precision Float(number=w363) -> (double precision float=w364:dbl[])
        n189 = To Double Precision Float(number=w361) -> (double precision float=w360:dbl[])
        n190 = To Double Precision Float(number=w362) -> (double precision float=w359:dbl[])
        n191 = Number To Fractional String(number=w337, precision (6)=w259) -> (F-format string=w345:string)  [unwired: 2 out]
        n192 = Number To Fractional String(number=w336, precision (6)=w259) -> (F-format string=w348:string)  [unwired: 2 out]
        n193 = Number To Fractional String(number=w320, precision (6)=w259) -> (F-format string=w330:string)  [unwired: 2 out]
        n194 = Number To Fractional String(number=w319, precision (6)=w259) -> (F-format string=w327:string)  [unwired: 2 out]
        n195 = Array To Spreadsheet String(array=w340, 3:w254) -> (spreadsheet string=w352:string)  [unwired: 1 out]
        n196 = for {
          tunnel: w338 -> [w561] mode=indexing
          tunnel: w339 -> [w563] mode=indexing
          tunnel: [w562] -> w349 mode=indexing
          n197 = Insert Into Array(array=w561, index=0, new element=w563) -> (w562:dbl[])
        }
        n198 = Array To Spreadsheet String(array=w321, 3:w254) -> (spreadsheet string=w323:string)  [unwired: 1 out]
        n199 = for {
          tunnel: w318 -> [w556] mode=indexing
          tunnel: [w557] -> w326 mode=indexing
          tunnel: w317 -> [w555] mode=indexing
          n200 = Insert Into Array(array=w556, index=0, new element=w555) -> (w557:dbl[])
        }
        n201 = Number To Fractional String(number=w302, precision (6)=w259) -> (F-format string=w308:string)  [unwired: 2 out]
        n202 = Number To Fractional String(number=w301, precision (6)=w259) -> (F-format string=w311:string)  [unwired: 2 out]
        n203 = Number To Fractional String(number=w284, precision (6)=w259) -> (F-format string=w294:string)  [unwired: 2 out]
        n204 = Number To Fractional String(number=w283, precision (6)=w259) -> (F-format string=w291:string)  [unwired: 2 out]
        n205 = Array To Spreadsheet String(array=w303, 3:w254) -> (spreadsheet string=w315:string)  [unwired: 1 out]
        n206 = for {
          tunnel: w300 -> [w550] mode=indexing
          tunnel: [w551] -> w312 mode=indexing
          tunnel: w299 -> [w549] mode=indexing
          n207 = Insert Into Array(array=w550, index=0, new element=w549) -> (w551:dbl[])
        }
        n208 = Array To Spreadsheet String(array=w285, 3:w254) -> (spreadsheet string=w287:string)  [unwired: 1 out]
        n209 = for {
          tunnel: w282 -> [w544] mode=indexing
          tunnel: [w545] -> w290 mode=indexing
          tunnel: w281 -> [w543] mode=indexing
          n210 = Insert Into Array(array=w544, index=0, new element=w543) -> (w545:dbl[])
        }
        n211 = To Double Precision Float(number=w506) -> (double precision float=w358:dbl)
        n212 = Divide(x=w364, y=w358) -> (x/y=w357:dbl[])
        n213 = Divide(x=w360, y=w358) -> (x/y=w356:dbl[])
        n214 = Divide(x=w359, y=w358) -> (x/y=w355:dbl[])
        n215 = Format Into String(initial string="\t", w352) -> (resulting string=w346:string)  [unwired: 2 in, 1 out]
        n216 = Format Into String(initial string="\t", w323) -> (resulting string=w329:string)  [unwired: 2 in, 1 out]
        n217 = Format Into String(initial string="\t", w315) -> (resulting string=w309:string)  [unwired: 2 in, 1 out]
        n218 = Format Into String(initial string="\t", w287) -> (resulting string=w293:string)  [unwired: 2 in, 1 out]
        n219 = Build Path(base path=w265, name or relative path="pdf Tau.txt" ("string")) -> (appended path=w404:path)
        n220 = Build Path(base path=w265, name or relative path="pdf U sync'd.txt" ("string")) -> (appended path=w452:path)
        n221 = Build Path(base path=w265, name or relative path=w401) -> (appended path=w445:path)
        n222 = Build Path(base path=w265, name or relative path=w400) -> (appended path=w441:path)
        n223 = Divide(x=w501, y=w509) -> (x/y=w508:dbl[])
        n224 = Divide(x=w500, y=w358) -> (x/y=w507:dbl[])
        n225 = case shown="\"V\", Default" w246 {
          tunnel: ["UbinW_WbinW_2Ddata\n" ("initial string") "UbinW_VbinW_2Ddata\n" ("initial string")] -> w277
          frame "W" {
          }
          frame "V", Default {
          }
        }
        n226 = Build Array(w402, w407) -> (w405:dbl[][])
        n227 = Build Array(w413, w449) -> (w451:dbl[][])
        n228 = Build Array(w397, w448) -> (w446:dbl[][])
        n229 = Build Array(w416, w442) -> (w444:dbl[][])
        n230 = case shown="True" w335 {
          tunnel: ["hist." ("string") "pdf" ("string")] -> w365
          frame False {
          }
          frame True {
          }
        }
        n231 = Format Into String(initial string=w342, w343, w345, w343, w348, w343, w343) -> (resulting string=w344:string)  [unwired: 2 in, 1 out]
        n232 = Array To Spreadsheet String(array=w349, 3:w254) -> (spreadsheet string=w347:string)  [unwired: 1 out]
        n233 = Format Into String(initial string=w333, w332, w330, w332, w327, w332, w332) -> (resulting string=w331:string)  [unwired: 2 in, 1 out]
        n234 = Array To Spreadsheet String(array=w326, 3:w254) -> (spreadsheet string=w328:string)  [unwired: 1 out]
        n235 = Format Into String(initial string=w305, w306, w308, w306, w311, w306, w306) -> (resulting string=w307:string)  [unwired: 2 in, 1 out]
        n236 = Array To Spreadsheet String(array=w312, 3:w254) -> (spreadsheet string=w310:string)  [unwired: 1 out]
        n237 = Format Into String(initial string=w297, w296, w294, w296, w291, w296, w296) -> (resulting string=w295:string)  [unwired: 2 in, 1 out]
        n238 = Array To Spreadsheet String(array=w290, 3:w254) -> (spreadsheet string=w292:string)  [unwired: 1 out]
        n239 = case shown="True" w335 {
          tunnel: [w587 w589] -> w369
          tunnel: w357 -> [w587 w590]
          tunnel: w354 -> [_ w594]
          frame False {
          }
          frame True {
            n240 = Index Array(array=w594, index=1) -> (element=w592:dbl)
            n241 = Index Array(array=w594, index=0) -> (element=w591:dbl)
            n242 = Subtract(x=w592, y=w591) -> (x-y=w588:dbl)
            n243 = Divide(x=w590, y=w588) -> (x/y=w589:dbl[])
          }
        }
        n244 = case shown="True" w335 {
          tunnel: [w578 w581] -> w370
          tunnel: w356 -> [w578 w582]
          tunnel: w280 -> [_ w579]
          frame False {
          }
          frame True {
            n245 = Index Array(array=w579, index=1) -> (element=w584:dbl)
            n246 = Index Array(array=w579, index=0) -> (element=w583:dbl)
            n247 = Subtract(x=w584, y=w583) -> (x-y=w580:dbl)
            n248 = Divide(x=w582, y=w580) -> (x/y=w581:dbl[])
          }
        }
        n249 = case shown="True" w335 {
          tunnel: [w569 w571] -> w376
          tunnel: w355 -> [w569 w572]
          tunnel: w279 -> [_ w576]
          frame False {
          }
          frame True {
            n250 = Index Array(array=w576, index=1) -> (element=w574:dbl)
            n251 = Index Array(array=w576, index=0) -> (element=w573:dbl)
            n252 = Subtract(x=w574, y=w573) -> (x-y=w570:dbl)
            n253 = Divide(x=w572, y=w570) -> (x/y=w571:dbl[])
          }
        }
        n254 = Transpose 2D Array(2D array=w405) -> (transposed array=w406:dbl[][])
        n255 = Transpose 2D Array(2D array=w451) -> (transposed array=w450:dbl[][])
        n256 = Transpose 2D Array(2D array=w446) -> (transposed array=w447:dbl[][])
        n257 = Transpose 2D Array(2D array=w444) -> (transposed array=w443:dbl[][])
        n258 = Build Path(base path=w265, name or relative path="2DPDF U - V sync'd.txt" ("string")) -> (appended path=w350:path)
        n259 = Concatenate Strings(w344, w346, w347) -> (w351:string)
        n260 = Build Path(base path=w265, name or relative path="2DPDF tau - U.txt" ("string")) -> (appended path=w325:path)
        n261 = Concatenate Strings(w331, w329, w328) -> (w324:string)
        n262 = Build Path(base path=w265, name or relative path="2DPDF tau - V.txt" ("string")) -> (appended path=w313:path)
        n263 = Concatenate Strings(w307, w309, w310) -> (w314:string)
        n264 = Build Path(base path=w265, name or relative path="2DPDF tau - UV.txt" ("string")) -> (appended path=w289:path)
        n265 = Concatenate Strings(w295, w293, w292) -> (w288:string)
        n266 = Array To Spreadsheet String(array=w406, 3:w254) -> (spreadsheet string=w411:string)  [unwired: 1 out]
        n267 = Array To Spreadsheet String(array=w450, 3:w254) -> (spreadsheet string=w437:string)  [unwired: 1 out]
        n268 = Array To Spreadsheet String(array=w447, 3:w254) -> (spreadsheet string=w431:string)  [unwired: 1 out]
        n269 = Array To Spreadsheet String(array=w443, 3:w254) -> (spreadsheet string=w426:string)  [unwired: 1 out]
        n270 = Number To Fractional String(number=w261, precision (6)=w259) -> (F-format string=w274:string)  [unwired: 2 out]
        n271 = Number To Fractional String(number=w260, precision (6)=w259) -> (F-format string=w271:string)  [unwired: 2 out]
        n272 = Array To Spreadsheet String(array=w264, 3:w254) -> (spreadsheet string=w267:string)  [unwired: 1 out]
        n273 = for {
          tunnel: w263 -> [w538] mode=indexing
          tunnel: [w539] -> w270 mode=indexing
          tunnel: w262 -> [w537] mode=indexing
          n274 = Insert Into Array(array=w538, index=0, new element=w537) -> (w539:dbl[])
        }
        n275 = Format Into String(initial string="binC" ("string"), "\t", w365, "\r", w431) -> (resulting string=w432:string)  [unwired: 2 in, 1 out]
        n276 = Format Into String(initial string="binC" ("string"), "\t", w365, "\r", w426) -> (resulting string=w427:string)  [unwired: 2 in, 1 out]
        n277 = Format Into String(initial string="binC" ("string"), "\t", w365, "\r", w411) -> (resulting string=w412:string)  [unwired: 2 in, 1 out]
        n278 = Format Into String(initial string="binC" ("string"), "\t", w365, "\r", w437) -> (resulting string=w436:string)  [unwired: 2 in, 1 out]
        n279 = Write to Text File(file (use dialog)=w350, text=w351) -> ()  [unwired: 1 in, 4 out]
        n280 = Write to Text File(file (use dialog)=w325, text=w324) -> ()  [unwired: 1 in, 4 out]
        n281 = Write to Text File(file (use dialog)=w313, text=w314) -> ()  [unwired: 1 in, 4 out]
        n282 = Write to Text File(file (use dialog)=w289, text=w288) -> ()  [unwired: 1 in, 4 out]
        n283 = Write to Text File(file (use dialog)=w404, text=w412) -> ()  [unwired: 1 in, 4 out]
        n284 = Write to Text File(file (use dialog)=w452, text=w436) -> ()  [unwired: 1 in, 4 out]
        n285 = Write to Text File(file (use dialog)=w445, text=w432) -> ()  [unwired: 1 in, 4 out]
        n286 = Write to Text File(file (use dialog)=w441, text=w427) -> ()  [unwired: 1 in, 4 out]
        n287 = Format Into String(initial string="\t", w267) -> (resulting string=w273:string)  [unwired: 2 in, 1 out]
        n288 = Build Path(base path=w265, name or relative path="pdf U orig.txt" ("string")) -> (appended path=w366:path)
        n289 = Build Path(base path=w265, name or relative path=w393) -> (appended path=w373:path)
        n290 = Build Path(base path=w265, name or relative path=w394) -> (appended path=w377:path)
        n291 = Build Array(w354, w369) -> (w367:dbl[][])
        n292 = Build Array(w280, w370) -> (w372:dbl[][])
        n293 = Build Array(w279, w376) -> (w374:dbl[][])
        n294 = Format Into String(initial string=w277, w276, w274, w276, w271, w276, w276) -> (resulting string=w275:string)  [unwired: 2 in, 1 out]
        n295 = Array To Spreadsheet String(array=w270, 3:w254) -> (spreadsheet string=w272:string)  [unwired: 1 out]
        n296 = Transpose 2D Array(2D array=w367) -> (transposed array=w368:dbl[][])
        n297 = Transpose 2D Array(2D array=w372) -> (transposed array=w371:dbl[][])
        n298 = Transpose 2D Array(2D array=w374) -> (transposed array=w375:dbl[][])
        n299 = Array To Spreadsheet String(array=w368, 3:w254) -> (spreadsheet string=w381:string)  [unwired: 1 out]
        n300 = Array To Spreadsheet String(array=w371, 3:w254) -> (spreadsheet string=w387:string)  [unwired: 1 out]
        n301 = Array To Spreadsheet String(array=w375, 3:w254) -> (spreadsheet string=w392:string)  [unwired: 1 out]
        n302 = Build Path(base path=w265, name or relative path="2DPDF U - V orig.txt" ("string")) -> (appended path=w269:path)
        n303 = Concatenate Strings(w275, w273, w272) -> (w268:string)
        n304 = Format Into String(initial string="binC" ("string"), "\t", w365, "\r", w387) -> (resulting string=w386:string)  [unwired: 2 in, 1 out]
        n305 = Format Into String(initial string="binC" ("string"), "\t", w365, "\r", w392) -> (resulting string=w391:string)  [unwired: 2 in, 1 out]
        n306 = Format Into String(initial string="binC" ("string"), "\t", w365, "\r", w381) -> (resulting string=w382:string)  [unwired: 2 in, 1 out]
        n307 = Write to Text File(file (use dialog)=w366, text=w382) -> ()  [unwired: 1 in, 4 out]
        n308 = Write to Text File(file (use dialog)=w373, text=w386) -> ()  [unwired: 1 in, 4 out]
        n309 = Write to Text File(file (use dialog)=w377, text=w391) -> ()  [unwired: 1 in, 4 out]
        n310 = Write to Text File(file (use dialog)=w269, text=w268) -> ()  [unwired: 1 in, 4 out]
      }
    }
    "Block time pulse checksums" <- w117
    "PW, LDA_U, V, UV phase plot" <- w145
    "LDA orig. and sync'd U,V phase plot" <- w144
    n311 = And Array Elements(Boolean array=w117) -> (logical AND=→"All checksums okay":bool)
    n312 = Increment(x=w114) -> (x+1=→"Lag time loop no.":i32)
    n313 = Concatenate Strings("PW lag time (s)", w171, w169, w171, "PW Us Vs U V", w171, w170, w171) -> (w173:string)
    n314 = case shown="True" w167 {
      tunnel: w173 -> [_ w183]
      tunnel: w166 -> [w180 w182]
      tunnel: [w180 w181] -> w168
      frame False {
      }
      frame True {
        n315 = Write to Text File(file (use dialog)=w182, text=w183) -> (refnum out=w181:refnum<file>)  [unwired: 1 in, 3 out]
      }
    }
    "PW lag time" <- w164
  }
  "Corr coeff. tau, U with PW lag time" <- w90
  "Corr coeff. tau, V with PW lag time" <- w89
  "Corr coeff. tau, UV with PW lag time" <- w88
  "Total sync'd points" <- w72
  "PW reverse flow factor" <- w73
  "PW timeout fraction" <- w71
  "PW TOFmin cutoff fraction" <- w70
  "Total pre-sync LDA points" <- w68
  n316 = Increment(x=w1) -> (x+1=→"Lag time loops to do":i32)
  n317 = Multiply(x=w76, y=w51) -> (x*y=w65:dbl[])
  "Rlag (m)" <- w65
  n318 = Build Array(w76, w65, w90, w89, w88) -> (w87:dbl[][])
  n319 = Insert Into Array(array=w61, index=w5, new element=w53) -> (w60:dbl[])
  n320 = Insert Into Array(array=w59, index=w5, new element=w52) -> (w58:dbl[])
  n321 = Insert Into Array(array=w56, index=w5, new element=w50) -> (w55:dbl[])
  n322 = Transpose 2D Array(2D array=w87) -> (transposed array=w86:dbl[][])
  n323 = Insert Into Array(array=w60, index=w5, new element=w62) -> (w57:dbl[])
  n324 = Insert Into Array(array=w58, index=w5, new element=w51) -> (w29:dbl[])
  n325 = Insert Into Array(array=w55, index=w5, new element=w49) -> (w21:dbl[])
  n326 = Array To Spreadsheet String(array=w86, 3:w66) -> (spreadsheet string=w84:string)  [unwired: 1 out]
  "tlag(s) Rlag(m) tauU tauV tauUV" <- w84
  n327 = Insert Into Array(array=w57, index=w5, new element=w54) -> (w6:dbl[])
  n328 = Insert Into Array(array=w6, index=w5, new element=w4) -> (w3:dbl[])
  n329 = Concatenate Strings("tlag(s) Rlag(m) tauU tauV tauUV", "\r", w84) -> (w83:string)
  n330 = Multiply(x=w12, y=w12) -> (x*y=w13:i32)
  n331 = case shown="True" "Write lagged correls. file?" {
    tunnel: w83 -> [_ w803]
    tunnel: w80 -> [_ w802]
    frame False {
    }
    frame True {
      n332 = Write to Text File(file (use dialog)=w802, text=w803) -> (refnum out=w801:refnum<file>)  [unwired: 1 in, 3 out]
      n333 = Close File(refnum=w801) -> ()  [unwired: 1 in, 2 out]
    }
  }
  n334 = Add(x=w13, y=4) -> (x+y=w14:i32)
  n335 = Add(x=w12, y=2) -> (x+y=w22:i32)
  n336 = Add(x=w12, y=2) -> (x+y=w26:i32)
  n337 = case shown="True" "Write raw numbers to file?" {
    tunnel: w79 -> [_ w804]
    frame False {
    }
    frame True {
      n338 = Close File(refnum=w804) -> ()  [unwired: 1 in, 2 out]
    }
  }
  n339 = Delete From Array(array=w3, index=w14) -> (array with subset deleted=w16:dbl[])  [unwired: 1 in, 1 out]
  n340 = Delete From Array(array=w29, index=w22) -> (array with subset deleted=w32:dbl[])  [unwired: 1 in, 1 out]
  n341 = Delete From Array(array=w21, index=w26) -> (array with subset deleted=w23:dbl[])  [unwired: 1 in, 1 out]
  n342 = Add(x=w12, y=4) -> (x+y=w19:i32)
  n343 = Delete From Array(array=w32, length=2, index=2) -> (array with subset deleted=→"Weighted stats":dbl[])  [unwired: 1 out]
  n344 = Delete From Array(array=w23, length=2, index=2) -> (array with subset deleted=→"Un-weighted stats":dbl[])  [unwired: 1 out]
  n345 = Delete From Array(array=w16, index=w19) -> (array with subset deleted=w15:dbl[])  [unwired: 1 in, 1 out]
  n346 = Delete From Array(array=w15, length=2, index=4) -> (array with subset deleted=→"Sync'd stats":dbl[])  [unwired: 1 out]
